vi "UDP Factory Wrapper.vi"(8 "error in (no error)":errorcluster, 10 "UDP settings":T1) -> (0 "error out":errorcluster, 3 "UDP out":refnum<class "UDP.lvclass">)   [LabVIEW 2018, in "Instrument Addon Scripting API.lvlib"]
uses:
  Instrument Addon Scripting API.lvlib
  Addon/Support Libraries/Protocols.lvlibp/UDP/UDP Settings.ctl
  Addon/Support Libraries/Protocols.lvlibp/UDP/UDP.lvclass
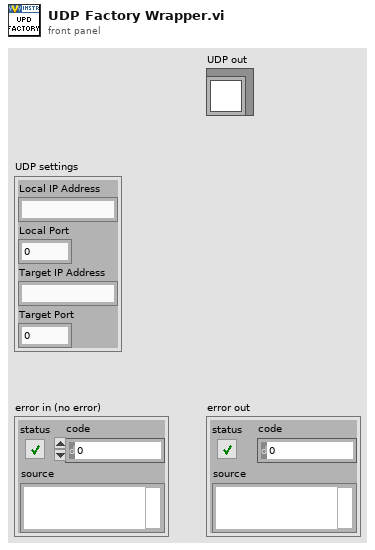
[diagram p1: front panel]
types:
  T1 = typedef "Protocols.lvlibp/UDP.lvclass/UDP Settings.ctl" = cluster{"Local IP Address":string, "Local Port":u16, "Target IP Address":string, "Target Port":u16}
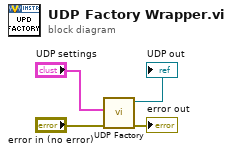
[diagram p0: block diagram]
diagram:
  n1 = call "UDP Factory.vi"("Error In"="error in (no error)", "UDP Settings"="UDP settings") -> ("Error Out"=→"error out":errorcluster, "UDP Out"=→"UDP out":refnum<class "UDP.lvclass">)  [unwired: 8 in]
